vi "Fetch Multi Eval Meas List Power Spectral Density Results.vi"(8 "error in (no error)":errorcluster, 9 "Result Type (Current)":i32(ring) items=["Current"=0, "Average"=1, "Standard Deviation"=3, "Maximum"=4, "Minimum"=5], 10 "Instance (1)":T1=1, 11 "VISA resource name":refnum<visa-resource-name>) -> (0 "error out":errorcluster, 1 "Results":dbl[](array[numeric]) format="%^.3e", 2 "Reliability":i32, 3 "VISA resource name out":refnum<visa-resource-name>)   [LabVIEW 2020, in "Rohde&Schwarz CMWXP NR FR1 Measurement.lvlib"]
doc: "Return RB power values (power spectral density) for all measured list mode segments.\n\nAttributes:\nRSCMWXPNRFR1M_ATTR_FETCH_MULTI_EVAL_MEAS_LIST_POWER_SPECTRAL_DENSITY_CURRENT_RESULTS\nRSCMWXPNRFR1M_ATTR_FETCH_MULTI_EVAL_MEAS_LIST_POWER_SPECTRAL_DENSITY_AVERAGE_RESULTS\nRSCMWXPNRFR1M_ATTR_FETCH_MULTI_EVAL_MEAS_LIST_POWER_SPECTRAL_DENSITY_STANDARD_DEVIATION_RESULTS\nRSCMWXPNRFR1M_ATTR_FETCH_MULTI_EVAL_MEAS_LIST_POWER_SPECTRAL_DENSITY_MAXIMUM_RESULTS\nRSCMWXPNRFR1M_ATTR_FETCH_MULTI_EVAL_MEAS_LIST_POWER_SPECTRAL_DENSITY_MINIMUM_RESULTS\n\nRemote-control commands:\nFETCh:NRSub:MEAS<i>:MEValuation:LIST:MODulation:PSD:CURRent?\nFETCh:NRSub:MEAS<i>:MEValuation:LIST:MODulation:PSD:AVERage?\nFETCh:NRSub:MEAS<i>:MEValuation:LIST:MODulation:PSD:SDEViation?\nFETCh:NRSub:MEAS<i>:MEValuation:LIST:MODulation:PSD:MAXimum?\nFETCh:NRSub:MEAS<i>:MEValuation:LIST:MODulation:PSD:MINimum?"
uses:
  <instrlib>/Rohde&Schwarz CMWXP NR FR1 Measurement/Rohde&Schwarz CMWXP NR FR1 Measurement.lvlib
  <instrlib>/Rohde&Schwarz CMWXP NR FR1 Measurement/Private/_Instance.ctl
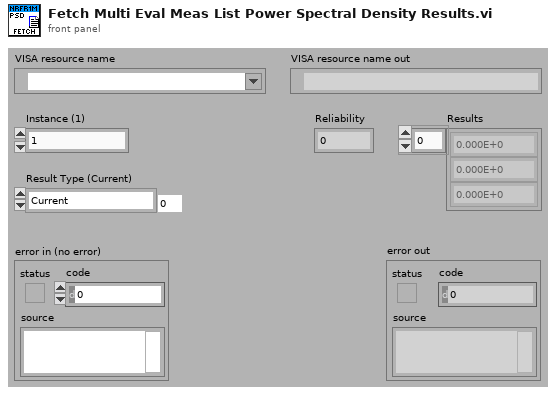
[diagram p1: front panel]
types:
  T1 = typedef "Rohde&Schwarz CMWXP NR FR1 Measurement.lvlib/_Instance.ctl" = i32
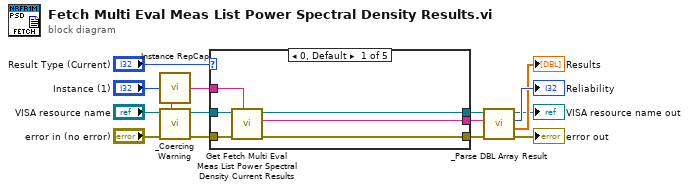
[diagram p0: block diagram]
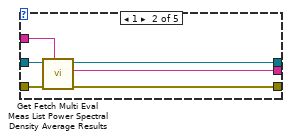
[diagram p2: hidden frame]
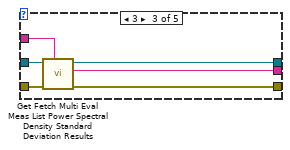
[diagram p3: hidden frame]
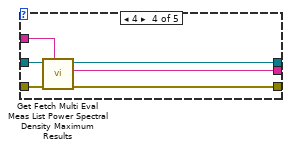
[diagram p4: hidden frame]
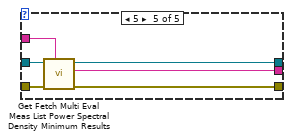
[diagram p5: hidden frame]
diagram:
  n1 = call <instrlib>:"Instance RepCap.vi"("Instance In"="Instance (1)") -> ("In Range?"=w13:bool, "RepCap Identifier Out"=w11:string)  [unwired: 1 in]
  n2 = call <instrlib>:"_Coercing Warning.vi"("In Range?"=w13, "error in (no error)"="error in (no error)", "VISA resource name"="VISA resource name") -> ("error out"=w9:errorcluster, "VISA resource name out"=w10:refnum<visa-resource-name>)  [unwired: 7 in]
  n3 = case shown="0, Default" "Result Type (Current)" {
    tunnel: w11 -> [w21 w27 w33 w39 w45]
    tunnel: w10 -> [w20 w26 w32 w38 w44]
    tunnel: w9 -> [w19 w25 w31 w37 w43]
    tunnel: [w18 w24 w30 w36 w42] -> w5
    tunnel: [w17 w23 w29 w35 w41] -> w6
    tunnel: [w16 w22 w28 w34 w40] -> w7
    frame 0, Default {
      n4 = call "Get Fetch Multi Eval Meas List Power Spectral Density Current Results"("Repeated Capabilities"=w21, "error in (no error)"=w19, "instrument handle"=w20) -> ("error out"=w16:errorcluster, "Fetch Multi Eval Meas List Power Spectral Density Current Results"=w17:string, "instrument handle out"=w18:refnum<visa-resource-name>)  [unwired: 6 in]
    }
    frame 1 {
      n5 = call "Get Fetch Multi Eval Meas List Power Spectral Density Average Results"("Repeated Capabilities"=w27, "error in (no error)"=w25, "instrument handle"=w26) -> ("error out"=w22:errorcluster, "Fetch Multi Eval Meas List Power Spectral Density Average Results"=w23:string, "instrument handle out"=w24:refnum<visa-resource-name>)  [unwired: 6 in]
    }
    frame 3 {
      n6 = call "Get Fetch Multi Eval Meas List Power Spectral Density Standard Deviation Results"("Repeated Capabilities"=w33, "error in (no error)"=w31, "instrument handle"=w32) -> ("error out"=w28:errorcluster, "Fetch Multi Eval Meas List Power Spectral Density Standard Deviation Results"=w29:string, "instrument handle out"=w30:refnum<visa-resource-name>)  [unwired: 6 in]
    }
    frame 4 {
      n7 = call "Get Fetch Multi Eval Meas List Power Spectral Density Maximum Results"("Repeated Capabilities"=w39, "error in (no error)"=w37, "instrument handle"=w38) -> ("error out"=w34:errorcluster, "Fetch Multi Eval Meas List Power Spectral Density Maximum Results"=w35:string, "instrument handle out"=w36:refnum<visa-resource-name>)  [unwired: 6 in]
    }
    frame 5 {
      n8 = call "Get Fetch Multi Eval Meas List Power Spectral Density Minimum Results"("Repeated Capabilities"=w45, "error in (no error)"=w43, "instrument handle"=w44) -> ("error out"=w40:errorcluster, "Fetch Multi Eval Meas List Power Spectral Density Minimum Results"=w41:string, "instrument handle out"=w42:refnum<visa-resource-name>)  [unwired: 6 in]
    }
  }
  n9 = call <instrlib>:"_Parse DBL Array Result.vi"("error in (no error)"=w7, "Input String"=w6, "VISA resource name"=w5) -> ("error out"=→"error out":errorcluster, "Results"=→"Results":dbl[], "Reliability"=→"Reliability":i32, "VISA resource name out"=→"VISA resource name out":refnum<visa-resource-name>)  [unwired: 5 in]
